vi "Decode DLL Output Codes SubVI.vi"(1 "Numeric":i32) -> (0 "Function Output Comment":string)   [LabVIEW 2015]
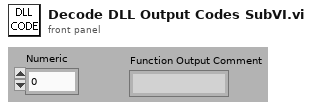
[diagram p1: front panel]
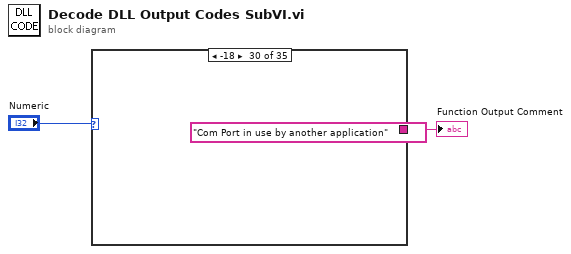
[diagram p0: block diagram]
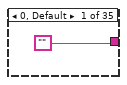
[diagram p2: hidden frame]
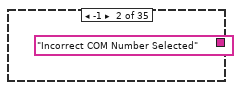
[diagram p3: hidden frame]
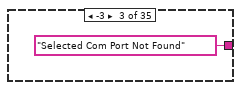
[diagram p4: hidden frame]
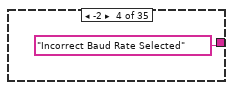
[diagram p5: hidden frame]
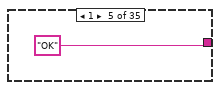
[diagram p6: hidden frame]
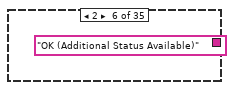
[diagram p7: hidden frame]
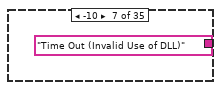
[diagram p8: hidden frame]
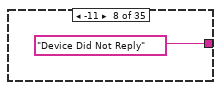
[diagram p9: hidden frame]
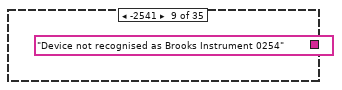
[diagram p10: hidden frame]
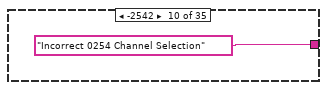
[diagram p11: hidden frame]
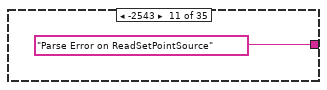
[diagram p12: hidden frame]
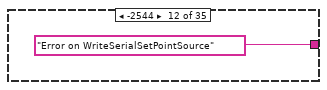
[diagram p13: hidden frame]
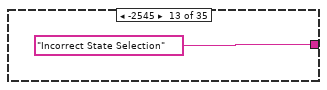
[diagram p14: hidden frame]
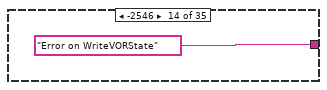
[diagram p15: hidden frame]
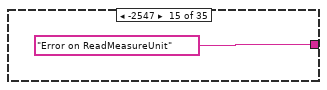
[diagram p16: hidden frame]
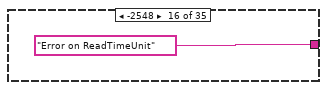
[diagram p17: hidden frame]
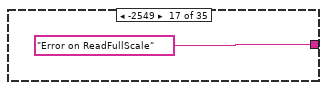
[diagram p18: hidden frame]
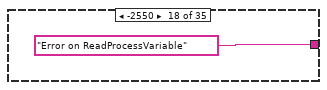
[diagram p19: hidden frame]
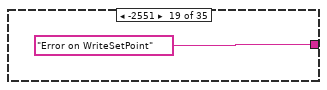
[diagram p20: hidden frame]
diagram:
  n1 = case shown="-18" "Numeric" {
    tunnel: ["" "Incorrect COM Number Selected" "Selected Com Port Not Found" "Incorrect Baud Rate Selected" "OK" "OK (Additional Status Available)" "Time Out (Invalid Use of DLL)" "Device Did Not Reply" "Device not recognised as Brooks Instrument 0254" "Incorrect 0254 Channel Selection" "Parse Error on ReadSetPointSource" "Error on WriteSerialSetPointSource" "Incorrect State Selection" "Error on WriteVORState" "Error on ReadMeasureUnit" "Error on ReadTimeUnit" "Error on ReadFullScale" "Error on ReadProcessVariable" "Error on WriteSetPoint" "Error on ReadSetPoint" "Error on ReadDecimalPlace" "Incorrect Decimal Place Selection" "Error on WriteDecimalPlace " "VOR State Out of Bounds (0, 1, or 2)" "Totalizer State Out of Bounds (0, 1, or 2)" "COMs Error" "CheckSum Error on COMs Error Message" "Incorrect Drop Type (0=SingleDrop; 1= MultiDrop)" "GasNumber Out of Range" "Com Port in use by another application" "Error at Set SetPoint" "Selected SetPointCode Incorrect" "Checksum Error in Reply" "Incorrect Byte Count in Reply" "TAG Number Wrong Length"] -> w2
    frame 0, Default {
    }
    frame -1 {
    }
    frame -3 {
    }
    frame -2 {
    }
    frame 1 {
    }
    frame 2 {
    }
    frame -10 {
    }
    frame -11 {
    }
    frame -2541 {
    }
    frame -2542 {
    }
    frame -2543 {
    }
    frame -2544 {
    }
    frame -2545 {
    }
    frame -2546 {
    }
    frame -2547 {
    }
    frame -2548 {
    }
    frame -2549 {
    }
    frame -2550 {
    }
    frame -2551 {
    }
    frame -2552 {
    }
    frame -2553 {
    }
    frame -2554 {
    }
    frame -2555 {
    }
    frame -12 {
    }
    frame -13 {
    }
    frame -14 {
    }
    frame -15 {
    }
    frame -16 {
    }
    frame -17 {
    }
    frame -18 {
    }
    frame -8 {
    }
    frame -7 {
    }
    frame -6 {
    }
    frame -5 {
    }
    frame -4 {
    }
  }
  "Function Output Comment" <- w2
